vi "Console_Write.vi"(10 "Code":string, 11 "Queue in":refnum<queue>) -> ()   [LabVIEW 2022 SP3]
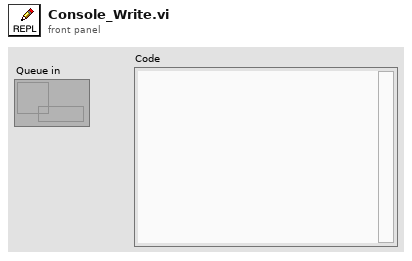
[diagram p1: front panel]
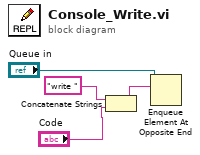
[diagram p0: block diagram]
diagram:
  n1 = Concatenate Strings("write " ("element"), "Code") -> (w3:string)
  n2 = Enqueue Element At Opposite End(queue="Queue in", element=w3) -> ()  [unwired: 2 in, 3 out]
